vi "find chapter test (FailsReport) (SubVI).vi"(0 "ForLoopIndex":i32, 1 "Fails ATR IN":string[][](array[string]), 2 "Full ATR":string[][](array[string]), 3 "FailsATR Index IN":i32, 5 "ToExecute?":bool, 6 "Fails ATR RowHeader IN":string[](array[string]), 8 "Full ATR RowHeader":string[](array[string])) -> (15 "Fails ATR OUT":string[][](array[string]), 16 "Fails ATR RowHeader OUT":string[](array[string]), 17 "FailsATR Index OUT":i32, 19 "ToExecute? Out":bool)   [LabVIEW 2017]
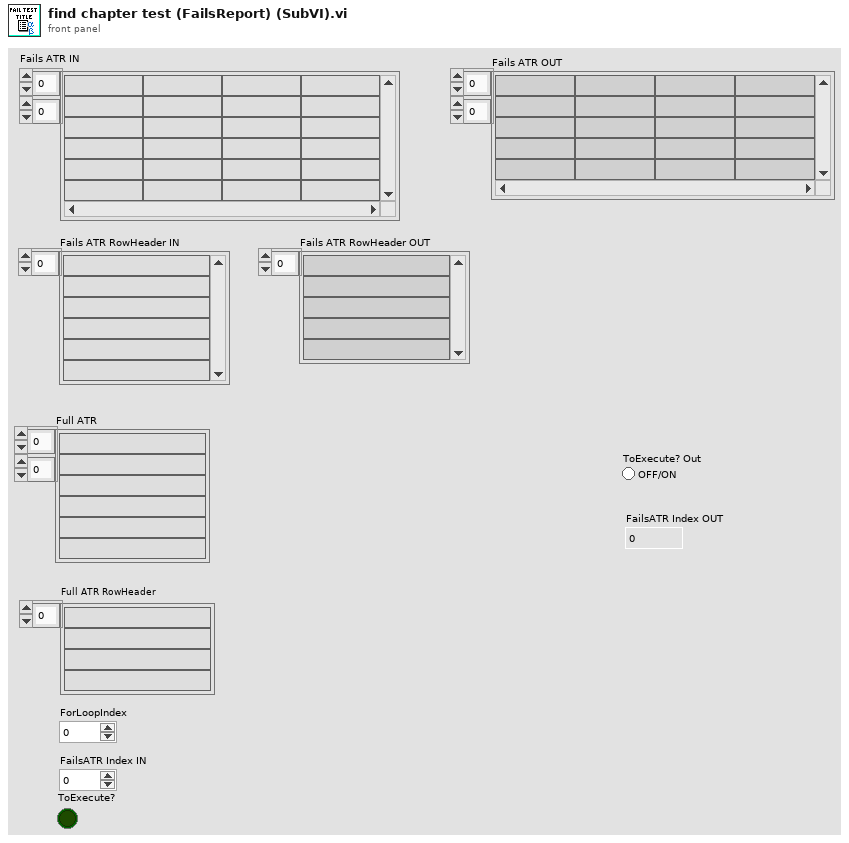
[diagram p1: front panel]
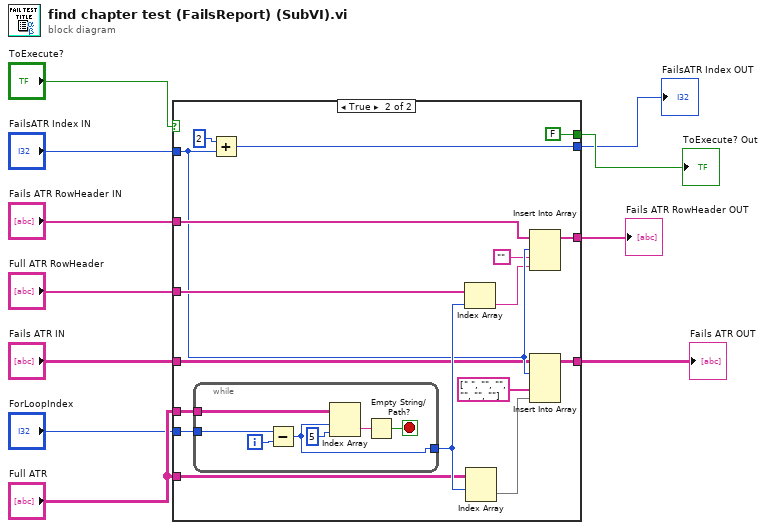
[diagram p0: block diagram]
diagram:
  n1 = case shown="True" "ToExecute?" {
    selector: "ToExecute?" -> [w15 _]
    tunnel: [w15 FALSE] -> w10
    tunnel: "Full ATR RowHeader" -> [_ w30]
    tunnel: "Fails ATR RowHeader IN" -> [w12 w29]
    tunnel: "FailsATR Index IN" -> [w13 w28]
    tunnel: "Fails ATR IN" -> [w14 w27]
    tunnel: "Full ATR" -> [_ w26]
    tunnel: "Full ATR" -> [_ w25]
    tunnel: "ForLoopIndex" -> [_ w24]
    tunnel: [w12 w23] -> w3
    tunnel: [w14 w22] -> w2
    tunnel: [w13 w21] -> w1
    frame False {
    }
    frame True {
      n2 = while {
        tunnel: [w36] -> w32
        tunnel: w25 -> [w34]
        tunnel: w24 -> [w33]
        i -> [w39]
        stop <- w35 stop-if-true
        n3 = Subtract(x=w33, y=w39) -> (x-y=w36:i32)
        n4 = Index Array(array=w34, index (row)=w36, index (col)=5 ("disabled index (col)")) -> (element=w37:string)
        n5 = Empty String/Path?(string/path=w37) -> (empty?=w35:bool)
      }
      n6 = Add(x=2, y=w28) -> (x+y=w21:i32)
      n7 = Index Array(array=w30, index=w32) -> (element=w17:string)
      n8 = Index Array(array=w26, index (row)=w32) -> (element=w19:string[])  [unwired: 1 in]
      n9 = Insert Into Array(array=w29, index=w28, new element #1="" ("new element/subarray"), new element #2=w17) -> (w23:string[])
      n10 = Insert Into Array(array=w27, index (row)=w28, new element #1=string[] [" ", "", "", "", "", ""] ("new element/subarray"), new element #2=w19) -> (w22:string[][])  [unwired: 1 in]
    }
  }
  "ToExecute? Out" <- w10
  "FailsATR Index OUT" <- w1
  "Fails ATR OUT" <- w2
  "Fails ATR RowHeader OUT" <- w3
